vi "Simple TCP - Server - 1.vi"() -> ()   [LabVIEW 2015]
doc: "Demonstrates how to set up a basic TCP connection, send data to the specified port once a connection has been established, and terminate the connection once the data has been sent. This VI is designed to stop if the TCP connection is terminated. The data sent in this example is an array of random numbers."
uses:
  <vilib>/Platform/TimedLoop/XDataNode/timing_clust.ctl
  <vilib>/Platform/TimedLoop/XDataNode/nitl_modes.ctl
  <vilib>/Platform/TimedLoop/XDataNode/wakeup.ctl
  <vilib>/platform/TimedLoop/XDataNode/XDataNode.xnode
  <vilib>/Platform/TimedLoop/XDataNode/XDNodeRunTimeDep.lvlib
panel:
  out "Time":u32
  out "Tries":i32
  out "Average Delay (ms)":dbl
  out "Delay (ms)":u32
  out "output cluster":T1
  in  "Client Closed":string="The client VI closed the connection."
  in  "Stop":bool
  # "Overview: Demonstrates the use of the TCP functions to initialize a TCP server that can send data to a client VI.\nInstructions:\n1. Run the VI.\n2. Open Simple TCP - Client.vi and follow the instructions on its front panel. Note that if you wait longer than 30 seconds to do this after running this VI, it will time out.\n3. Click Stop to stop the VI. Note that if you stop the client VI, this VI will stop automatically."
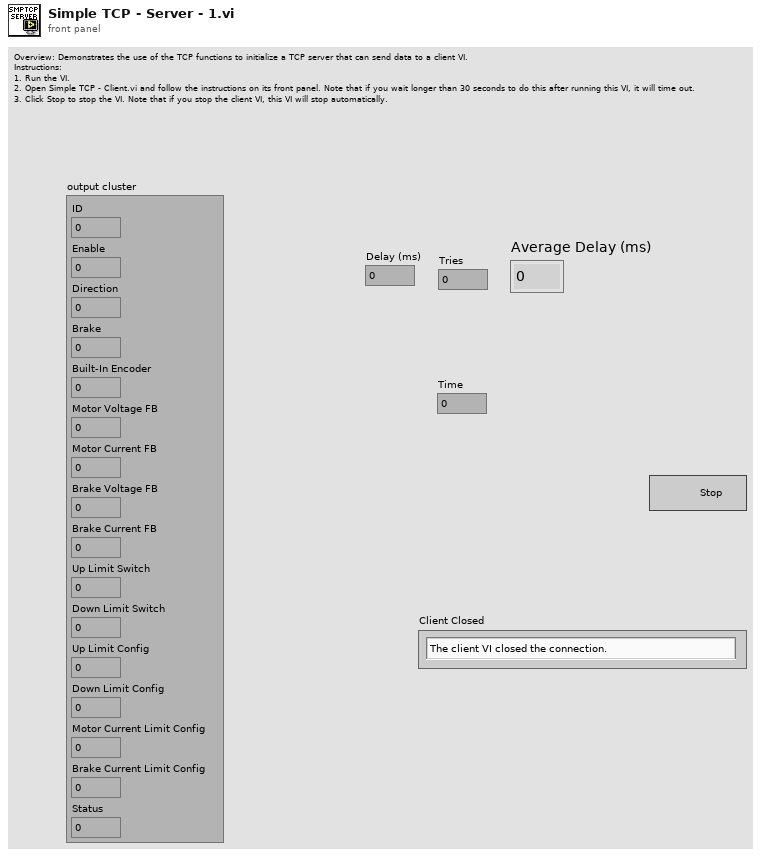
[diagram p1: front panel]
types:
  T1 = cluster{"ID":dbl, "Enable":dbl, "Direction":dbl, "Brake":dbl, "Built-In Encoder":dbl, "Motor Voltage FB":dbl, "Motor Current FB":dbl, "Brake Voltage FB":dbl, "Brake Current FB":dbl, "Up Limit Switch":dbl, "Down Limit Switch":dbl, "Up Limit Config":dbl, "Down Limit Config":dbl, "Motor Current Limit Config":dbl, "Brake Current Limit Config":dbl, "Status":dbl}
  T2 = typedef "XDNodeRunTimeDep.lvlib/timing_clust.ctl" = cluster{"Expected End [f-1]":u64, "Actual End [f-1]":u64, "Finished Late? [f-1]":bool, "Expected End [i-1]":u64, "Actual End [i-1]":u64, "Finished Late? [i-1]":bool, "Expected Start [i]":u64, "Actual Start [i]":u64, "Expected Start [f]":u64, "Actual Start [f]":u64, "Source Name":string, "Structure Name":string, "Period":i64, "Deadline":i64, "Offset":i64, "Start":i64, "Priority":i32, "Timeout":i32, "Mode":T3, "Wakeup Reason":T4, "Error":errorcluster, "Source Type":string, "Secondary Source Type":string, "Global End Time":u64, "Global Start Time":u64, "Frame Duration":u64, "Iteration Duration":u64, "Assigned CPU":i32, "I/O Scan Engine Mode":u32}
  T3 = typedef "XDNodeRunTimeDep.lvlib/nitl_modes.ctl" = enum32{"No Change", "Process missed periods, maintain original phase", "Discard missed periods, maintain original phase", "Process missed periods, ignore original phase", "Discard missed periods, ignore original phase"}
  T4 = typedef "XDNodeRunTimeDep.lvlib/wakeup.ctl" = enum32{"Normal", "Aborted", "Asynchronous wakeup", "Timing source error", "Timed loop error", "Timeout"}
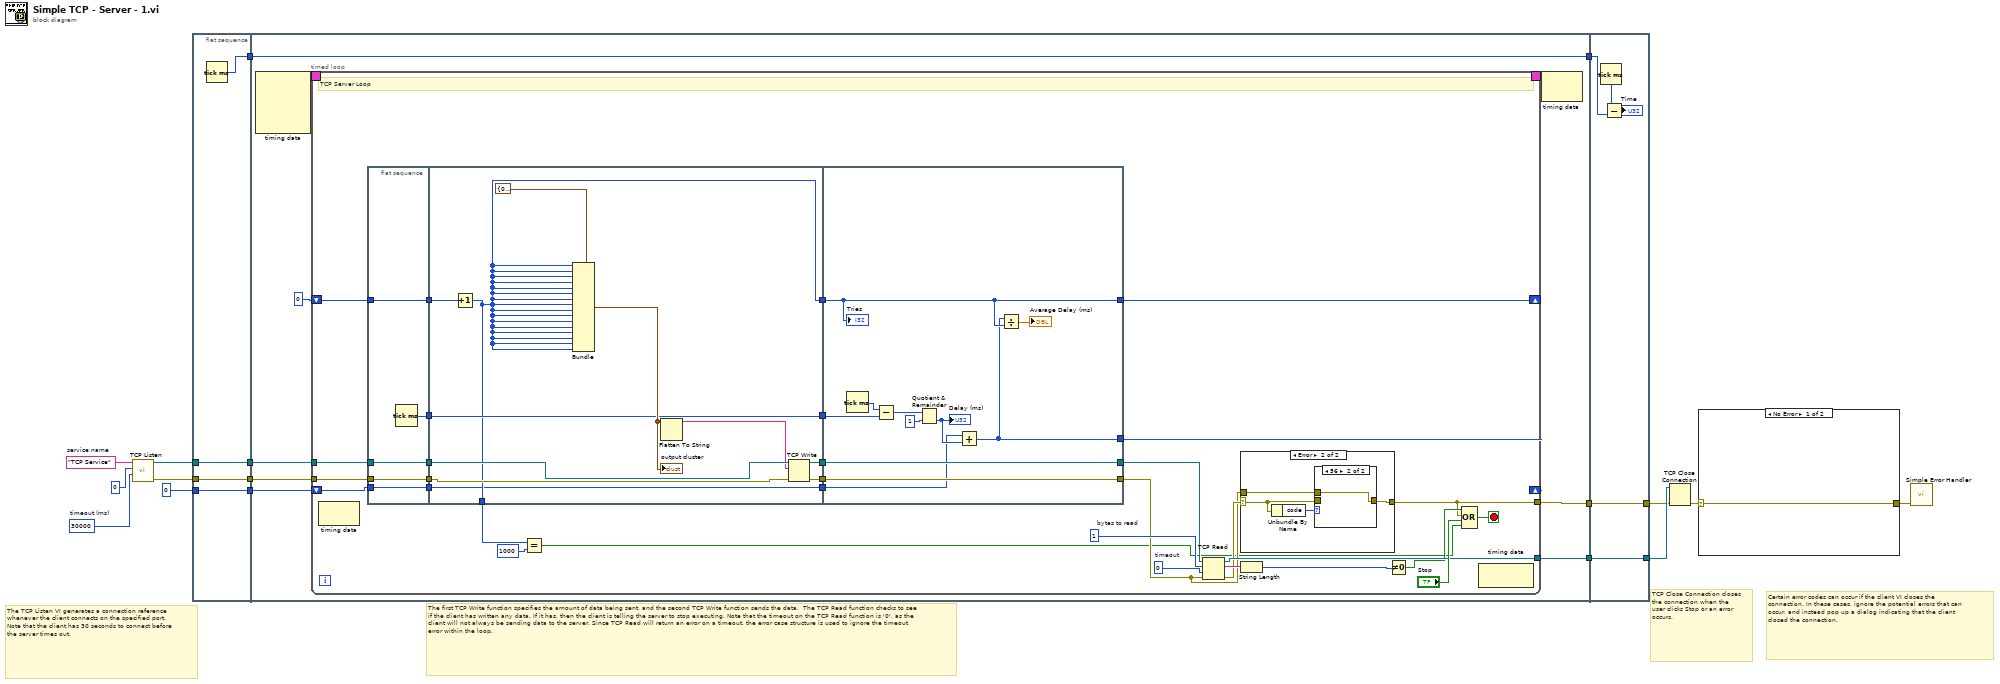
[diagram p0: block diagram]
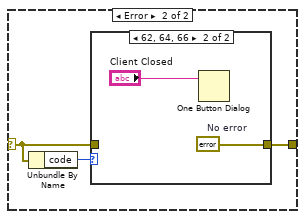
[diagram p4: hidden frame]
diagram:
  w10 = "TCP Service"  # service name
  w11 = 30000  # timeout (ms)
  # "TCP Close Connection closes the connection when the user clicks Stop or an error occurs."
  # "The TCP Listen VI generates a connection reference whenever the client connects on the specified port. Note that the client has 30 seconds to connect before the server times out."
  # "Certain error codes can occur if the client VI closes the connection. In these cases, ignore the potential errors that can occur, and instead pop up a dialog indicating that the client closed the connection."
  # "The first TCP Write function specifies the amount of data being sent, and the second TCP Write function sends the data.  The TCP Read function checks to see if the client has written any data. If it has, then the client is telling the server to stop executing. Note that the timeout on the TCP Read function is '0', as the client will not always be sending data to the server. Since TCP Read will return an error on a timeout, the error case structure is used to ignore the timeout error within the loop."
  n1 = call <vilib>:"TCP Listen.vi"("timeout ms (wait forever: -1)"=w11, "port"=u16 0, "service name"=w10) -> ("error out"=w12:errorcluster, "connection ID"=w13:refnum<k5>)  [unwired: 4 in, 3 out]
  n2 = flat-sequence {
    tunnel: 0 -> [w19]
    tunnel: w12 -> [w20]
    tunnel: w13 -> [w21]
    tunnel: [w21] -> w5
    tunnel: [w20] -> w4
    tunnel: [w19] -> w3
    tunnel: [w18] -> w1
    tunnel: [w28] -> w7
    tunnel: [w27] -> w6
    tunnel: w5 -> [w26]
    tunnel: w4 -> [w25]
    tunnel: w3 -> [w23]
    tunnel: [w22] -> w2
    tunnel: w1 -> [w22]
    tunnel: [w103] -> w16
    tunnel: [w104] -> w17
    tunnel: w7 -> [w104]
    tunnel: w6 -> [w103]
    tunnel: w2 -> [w101]
    frame #0 {
      n3 = Tick Count (ms)() -> (millisecond timer value=w18:u32)
    }
    frame #1 {
      n4 = node-c288() -> (w30:T2)  [unwired: 4 in]
      n5 = timed-loop {
        tunnel: [w49] -> w27
        tunnel: [w55] -> w28
        tunnel: w26 -> [w61]
        tunnel: w25 -> [w59]
        timing: w30 -> [_]
        timing-out: [_] -> w29
        shift-right: [w36] -> _
        shift-left: 0 -> [w38]
        shift-right: [w31] -> _
        shift-left: w23 -> [w32]
        stop <- w60 stop-if-true
        w54 = 0  # timeout
        w57 = 1  # bytes to read
        # "TCP Server Loop"
        n6 = node-c288() -> ()  [unwired: 1 in, 1 out]
        n7 = flat-sequence {
          tunnel: w59 -> [w65]
          tunnel: w61 -> [w66]
          tunnel: [w66] -> w43
          tunnel: [w65] -> w42
          tunnel: [w64] -> w40
          tunnel: [w63] -> w39
          tunnel: w38 -> [w63]
          tunnel: [w62] -> w33
          tunnel: w32 -> [w62]
          tunnel: [w75] -> w45
          tunnel: [w74] -> w44
          tunnel: w43 -> [w77]
          tunnel: w42 -> [w76]
          tunnel: [w70] -> w41
          tunnel: w40 -> [w70]
          tunnel: w39 -> [w69]
          tunnel: [w68] -> w37
          tunnel: [w68] -> w35
          tunnel: [w67] -> w34
          tunnel: w33 -> [w67]
          tunnel: [w87] -> w48
          tunnel: [w88] -> w56
          tunnel: w45 -> [w88]
          tunnel: w44 -> [w87]
          tunnel: w41 -> [w85]
          tunnel: [w81] -> w36
          tunnel: w35 -> [w81]
          tunnel: w34 -> [w80]
          tunnel: [w79] -> w31
          frame #0 {
            n8 = Tick Count (ms)() -> (millisecond timer value=w64:u32)
          }
          frame #1 {
            n9 = Increment(x=w69) -> (x+1=w68:i32)
            n10 = Bundle(cluster=T1 {"ID"=0.0, "Enable"=0.0, "Direction"=0.0, "Brake"=0.0, "Built-In Encoder"=0.0, "Motor Voltage FB"=0.0, "Motor Current FB"=0.0, "Brake Voltage FB"=0.0, "Brake Current FB"=0.0, "Up Limit Switch"=0.0, "Down Limit Switch"=0.0, "Up Limit Config"=0.0, "Down Limit Config"=0.0, "Motor Current Limit Config"=0.0, "Brake Current Limit Config"=0.0, "Status"=0.0} ("MirrorCoverMotor"), "ID"=w68, "Enable"=w68, "Direction"=w68, "Brake"=w68, "Built-In Encoder"=w68, "Motor Voltage FB"=w68, "Motor Current FB"=w68, "Brake Voltage FB"=w68, "Brake Current FB"=w68, "Up Limit Switch"=w68, "Down Limit Switch"=w68, "Up Limit Config"=w68, "Down Limit Config"=w68, "Motor Current Limit Config"=w68, "Brake Current Limit Config"=w68, "Status"=w68) -> (w73:T1)
            "output cluster" <- w73
            n11 = Flatten To String(anything=w73) -> (data string=w71:string)  [unwired: 3 in, 2 out]
            n12 = TCP Write(connection ID=w77, data in=w71, error in (no error)=w76) -> (connection ID out=w75:refnum<k5>, error out=w74:errorcluster)  [unwired: 2 out]
          }
          frame #2 {
            n13 = Tick Count (ms)() -> (millisecond timer value=w86:u32)
            n14 = Subtract(x=w86, y=w85) -> (x-y=w78:u32)
            n15 = Quotient & Remainder(x=w78, y=u32 1) -> (floor(x/y)=w83:u32)  [unwired: 1 out]
            "Delay (ms)" <- w83
            n16 = Add(x=w80, y=w83) -> (x+y=w79:u32)
            n17 = Divide(x=w79, y=w81) -> (x/y=→"Average Delay (ms)":dbl)
            "Tries" <- w81
          }
        }
        n18 = Equal?(x=w37, y=1000) -> (x = y?=w46:bool)
        n19 = TCP Read(connection ID=w56, bytes to read=w57, error in (no error)=w48, 9:w54) -> (connection ID out=w55:refnum<k5>, data out=w52:string, error out=w50:errorcluster)  [unwired: 1 out]
        n20 = case shown="Error" w50 {
          selector: w50 -> [w91 w94]
          tunnel: [w91 w92] -> w49
          tunnel: w48 -> [_ w93]
          frame No Error {
          }
          frame Error {
            n21 = Unbundle By Name(w94) -> ("code"=w95:i32)
            n22 = case shown="56" w95 {
              tunnel: w94 -> [w96 _]
              tunnel: w93 -> [_ w97]
              tunnel: [w96 w97] -> w92
              frame Default {
              }
              frame 56 {
              }
            }
          }
        }
        n23 = String Length(string=w52) -> (length=w53:i32)
        n24 = Not Equal To 0?(x=w53) -> (x != 0?=w51:bool)
        n25 = Compound Arithmetic op=OR(w51, w49, "Stop", w46) -> (w60:bool)
        n26 = node-c288() -> ()  [unwired: 1 in, 1 out]
      }
      n27 = node-c288(w29) -> ()  [unwired: 1 out]
    }
    frame #2 {
      n28 = Tick Count (ms)() -> (millisecond timer value=w102:u32)
      n29 = Subtract(x=w102, y=w101) -> (x-y=→"Time":u32)
    }
  }
  n30 = TCP Close Connection(connection ID=w17, error in (no error)=w16) -> (error out=w15:errorcluster)  [unwired: 2 out]
  n31 = case shown="No Error" w15 {
    selector: w15 -> [w105 w107]
    tunnel: [w105 w106] -> w14
    frame No Error {
    }
    frame Error {
      n32 = Unbundle By Name(w107) -> ("code"=w108:i32)
      n33 = case shown="62, 64, 66" w108 {
        tunnel: w107 -> [w109 _]
        tunnel: [w109 w111] -> w106
        frame Default {
        }
        frame 62, 64, 66 {
          w111 = errorcluster {"status"=FALSE, "code"=0, "source"=""}  # No error
          n34 = One Button Dialog(message="Client Closed") -> ()  [unwired: 1 in, 1 out]
        }
      }
    }
  }
  n35 = call <vilib>:"Simple Error Handler.vi"("error in (no error)"=w14) -> ()  [unwired: 1 in, 8 out]
